vi "final_usrp_transceiver_webcam.vi"() -> ()   [LabVIEW 2014]
uses:
  <vilib>/userdefined/High Color/IMAQdx.ctl
  <vilib>/addons/Modulation/Analog/support/mod_Set Error Source.vi
  var_stop.vi
  <vilib>/addons/Modulation/Digital/Support/Common/Validators/mod_Generate Filter Coefficients Validate.vi
  <vilib>/addons/Modulation/Digital/General/subVIs/mod_Generate Filter Coefficients.vi
  <vilib>/measure/maspectr.llb/FFT Power Spectrum and PSD for 1 Chan (CDB).vi
  <vilib>/addons/Modulation/Digital/General/MT Apply Matched Filter (Generic).vi
  <vilib>/addons/Modulation/Digital/General/MT Align to Ideal Symbols (Generic).vi
  <instrlib>/niUSRP/niUSRP Fetch Rx Data (CDB Cluster).vi
  <instrlib>/niUSRP/niUSRP Write Tx Data (CDB Cluster).vi
  <vilib>/addons/Modulation/Digital/General/MT Apply Pulse Shaping Filter (Generic).vi
  <vilib>/addons/Modulation/niDMT.lvlib
  <vilib>/measure/NI_MAPro.lvlib
  <vilib>/vision/driver/NI_Vision_Acquisition_Software.lvlib
panel:
  out "error out":errorcluster
  in  "cam":T1
  in  "frame buffer size":i32=20
  in  "Stop":bool
  in  "energy threshold":dbl=-33.0 format="%#_13g"
  out "elements in frame buffer 2":i32
  out "elements in frame buffer":i32
  out "valid frames":i32
  out "elements in send buffer":i32
  in  "packet size":i32=12800
  in  "Quality (0-1000)":i32=100 caption="Quality (750)"
  out "size(s) 4":i32
  out "frame num":u32
  out "length":i32[](array[numeric])
  out "start index":i32[](array[numeric])
  out "Numeric":i32
  out "size(s) 3":i32
  out "# elements in queue 2":i32
  out "size(s) 2":i32
  out "size(s)":i32[](array[numeric])
  out "image":T2(plugin-control)
  in  "Transmit power (db)":dbl
  out "found?":bool
  out "# elements in queue":i32
  out "valid?":bool
  in  "Gray code?":bool=TRUE
  in  "Modulation":enum16{"PSK", "QAM"}(ring)
  out "packet len":u32
  in  "filter length (symbols)":i32=8
  in  "filter parameter":dbl=0.5 format="%.2f"
  in  "pulse shaping filter (none)":T3(ring)=enum."Raised Cosine"
  in  "M-PSK (4)":i32=4 caption="M-ARY"
  in  "samples per symbol (16)":i32=4
  out "packet bits length":i32
  in  "number of samples":i64=40000
  out "RX coerced gain":dbl format="%#_6f"
  out "RX coerced carrier frequency":dbl=915000000.0 format="%#_6p"
  out "RX coerced IQ rate":dbl=4000000.0 format="%#_6p"
  in  "RX active antenna":string="RX2"
  in  "RX gain":dbl format="%#_6f"
  in  "RX device names":refnum<k15>="192.168.10.2"
  out "TX coerced gain":dbl format="%#_6f"
  out "TX coerced carrier frequency":dbl=915000000.0 format="%#_6p"
  out "coerced IQ rate":dbl=4000000.0 format="%#_6p"
  in  "TX device names":refnum<k15>="192.168.10.2"
  in  "TX gain":dbl format="%#_6f"
  in  "carrier frequency":dbl=915000000.0 format="%#_6p"
  in  "IQ rate":dbl=800000.0 format="%#_6p"
  in  "stop":bool
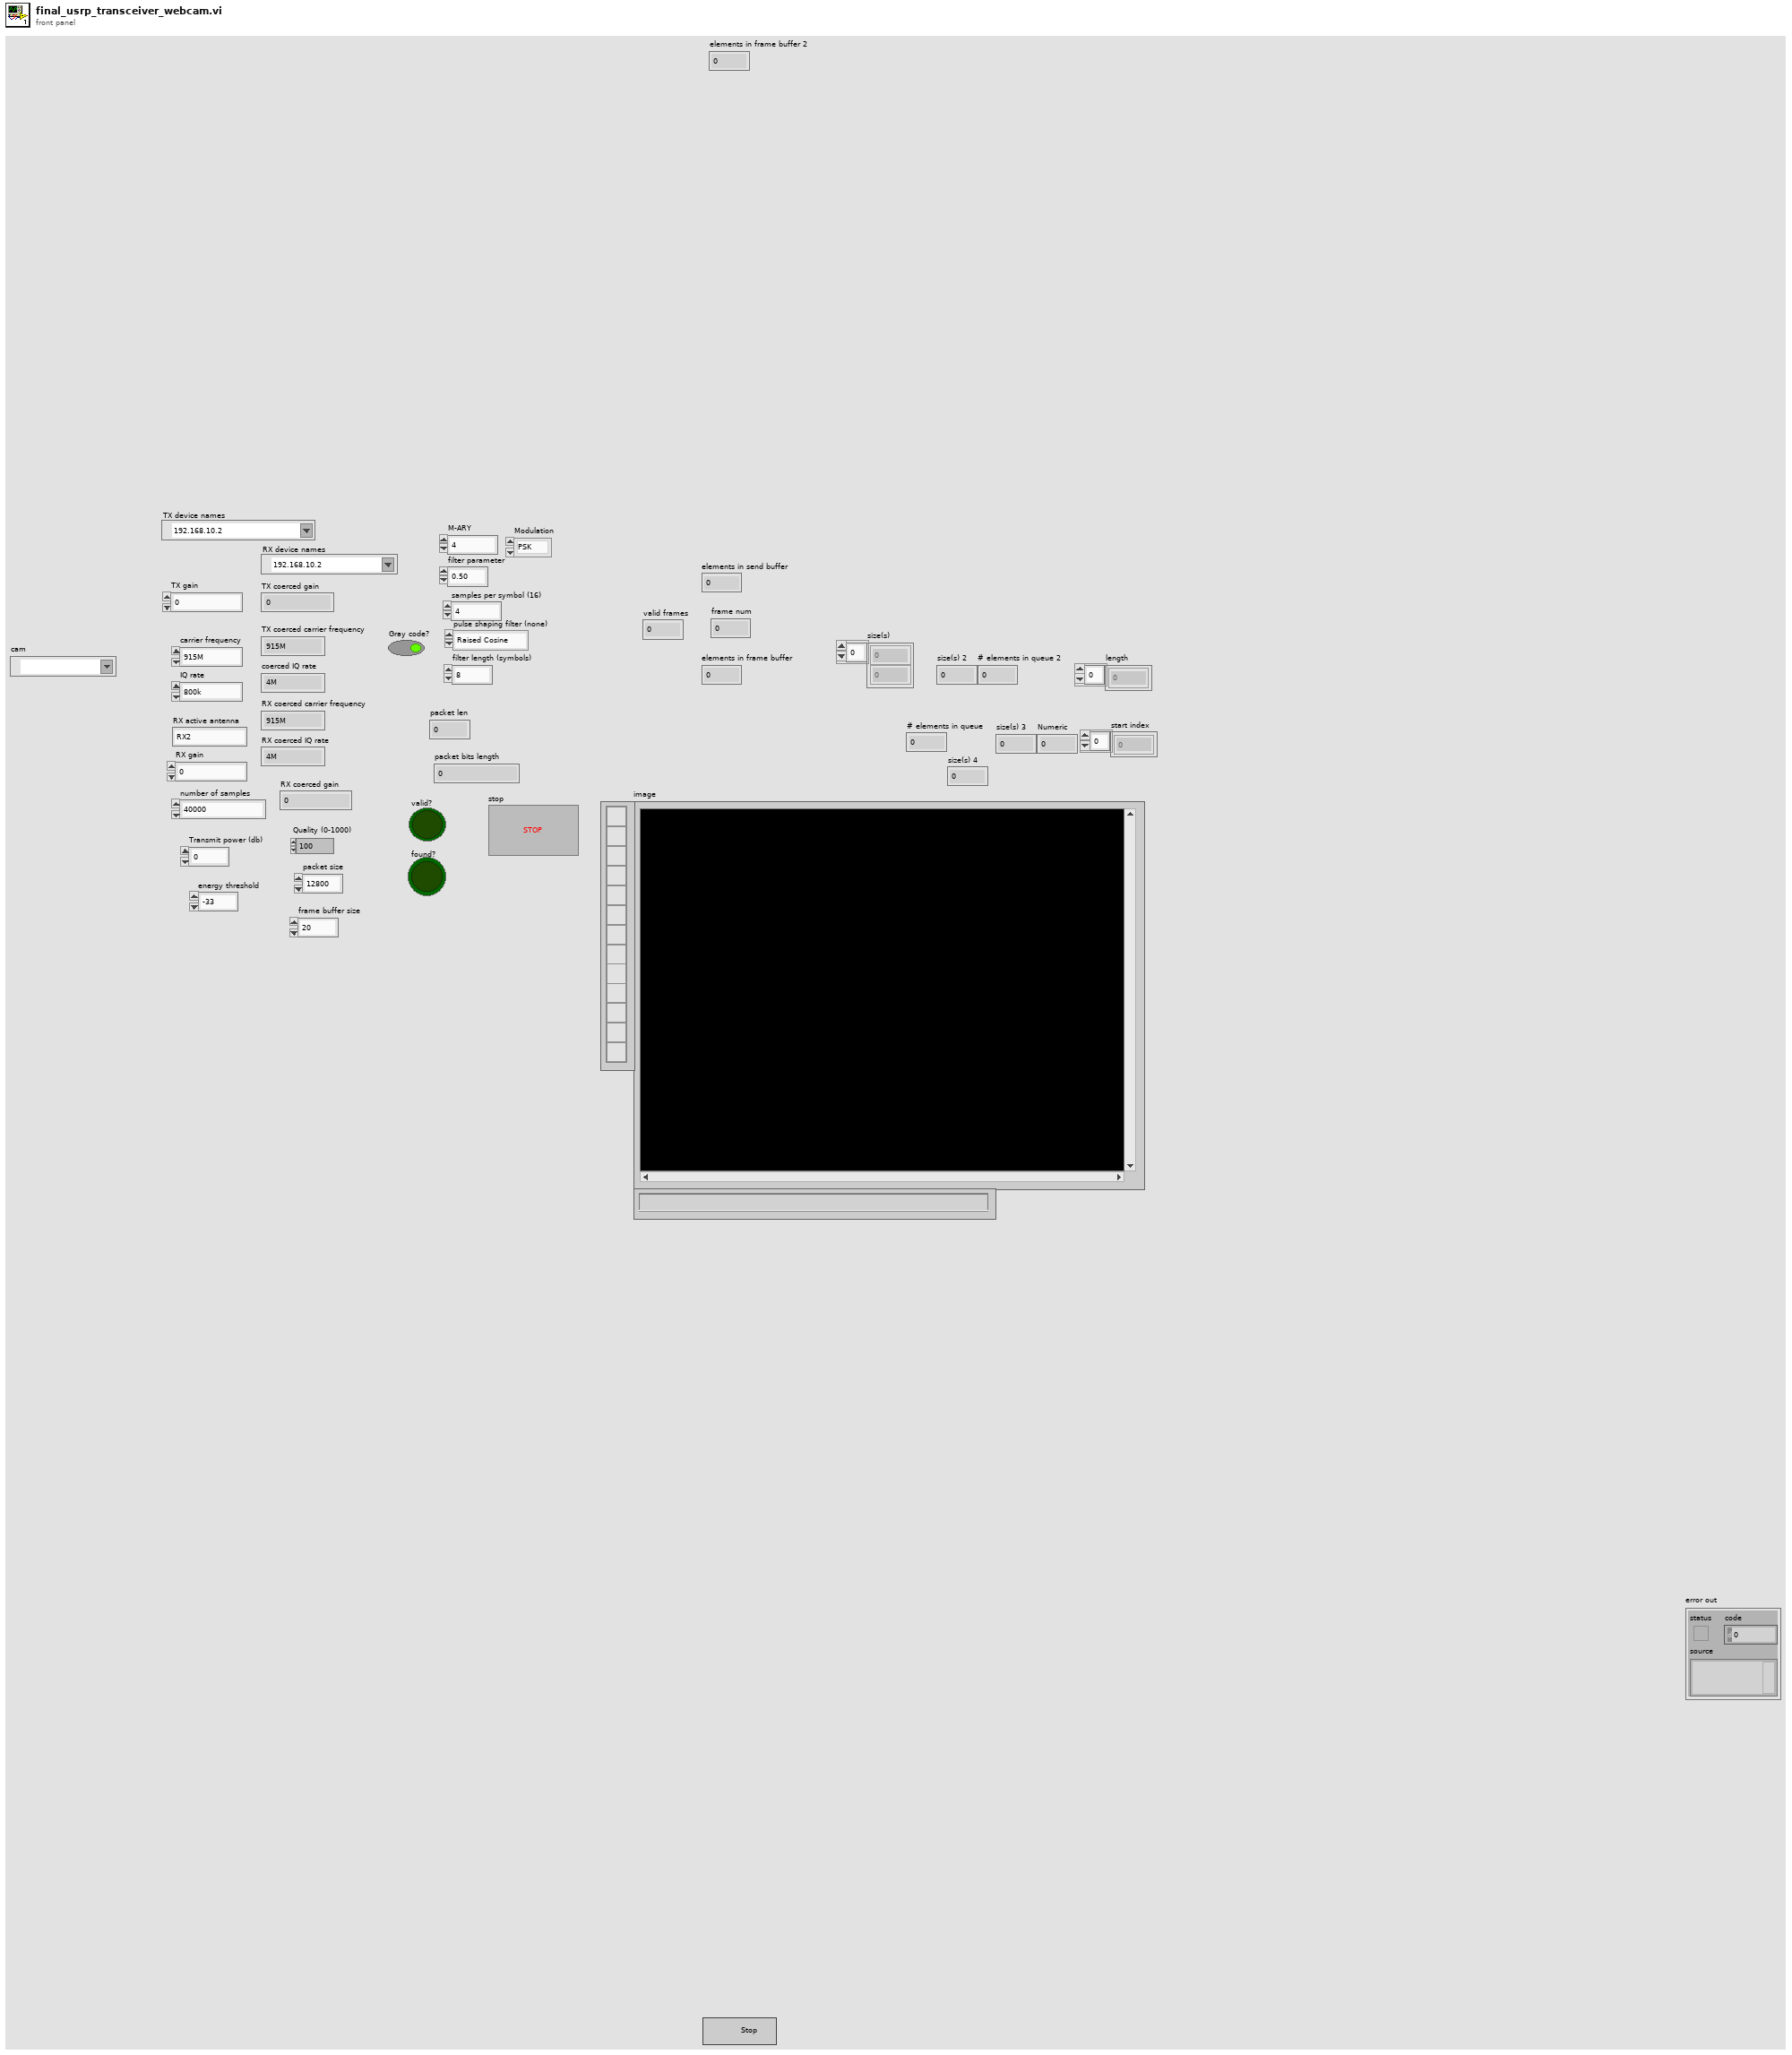
[diagram p1: front panel]
types:
  T1 = typedef "IMAQdx.ctl" = refnum<k21>
  T2 = typedef "IMAQ Image.ctl" = refnum<image>
  T3 = enum16{"none", "Raised Cosine", "Root Raised Cos", "Gaussian"}
  T4 = typedef "Image Type" = u32
  T5 = enum16{"FSK", "PSK", "QAM", "MSK", "PAM", "ASK", "CPM"}
  T6 = cluster{"samples per symbol (16)":i32, "symbol map":cdb[], "index map":u32[]}
  T7 = cluster{"samples per symbol (16)":i32, "symbol map":cdb[], i32[]}
  T8 = typedef "niAMT.lvlib/Complex Data Waveform.ctl" = cluster{"t0":dbl, "dt":dbl, "Y":cdb[]}
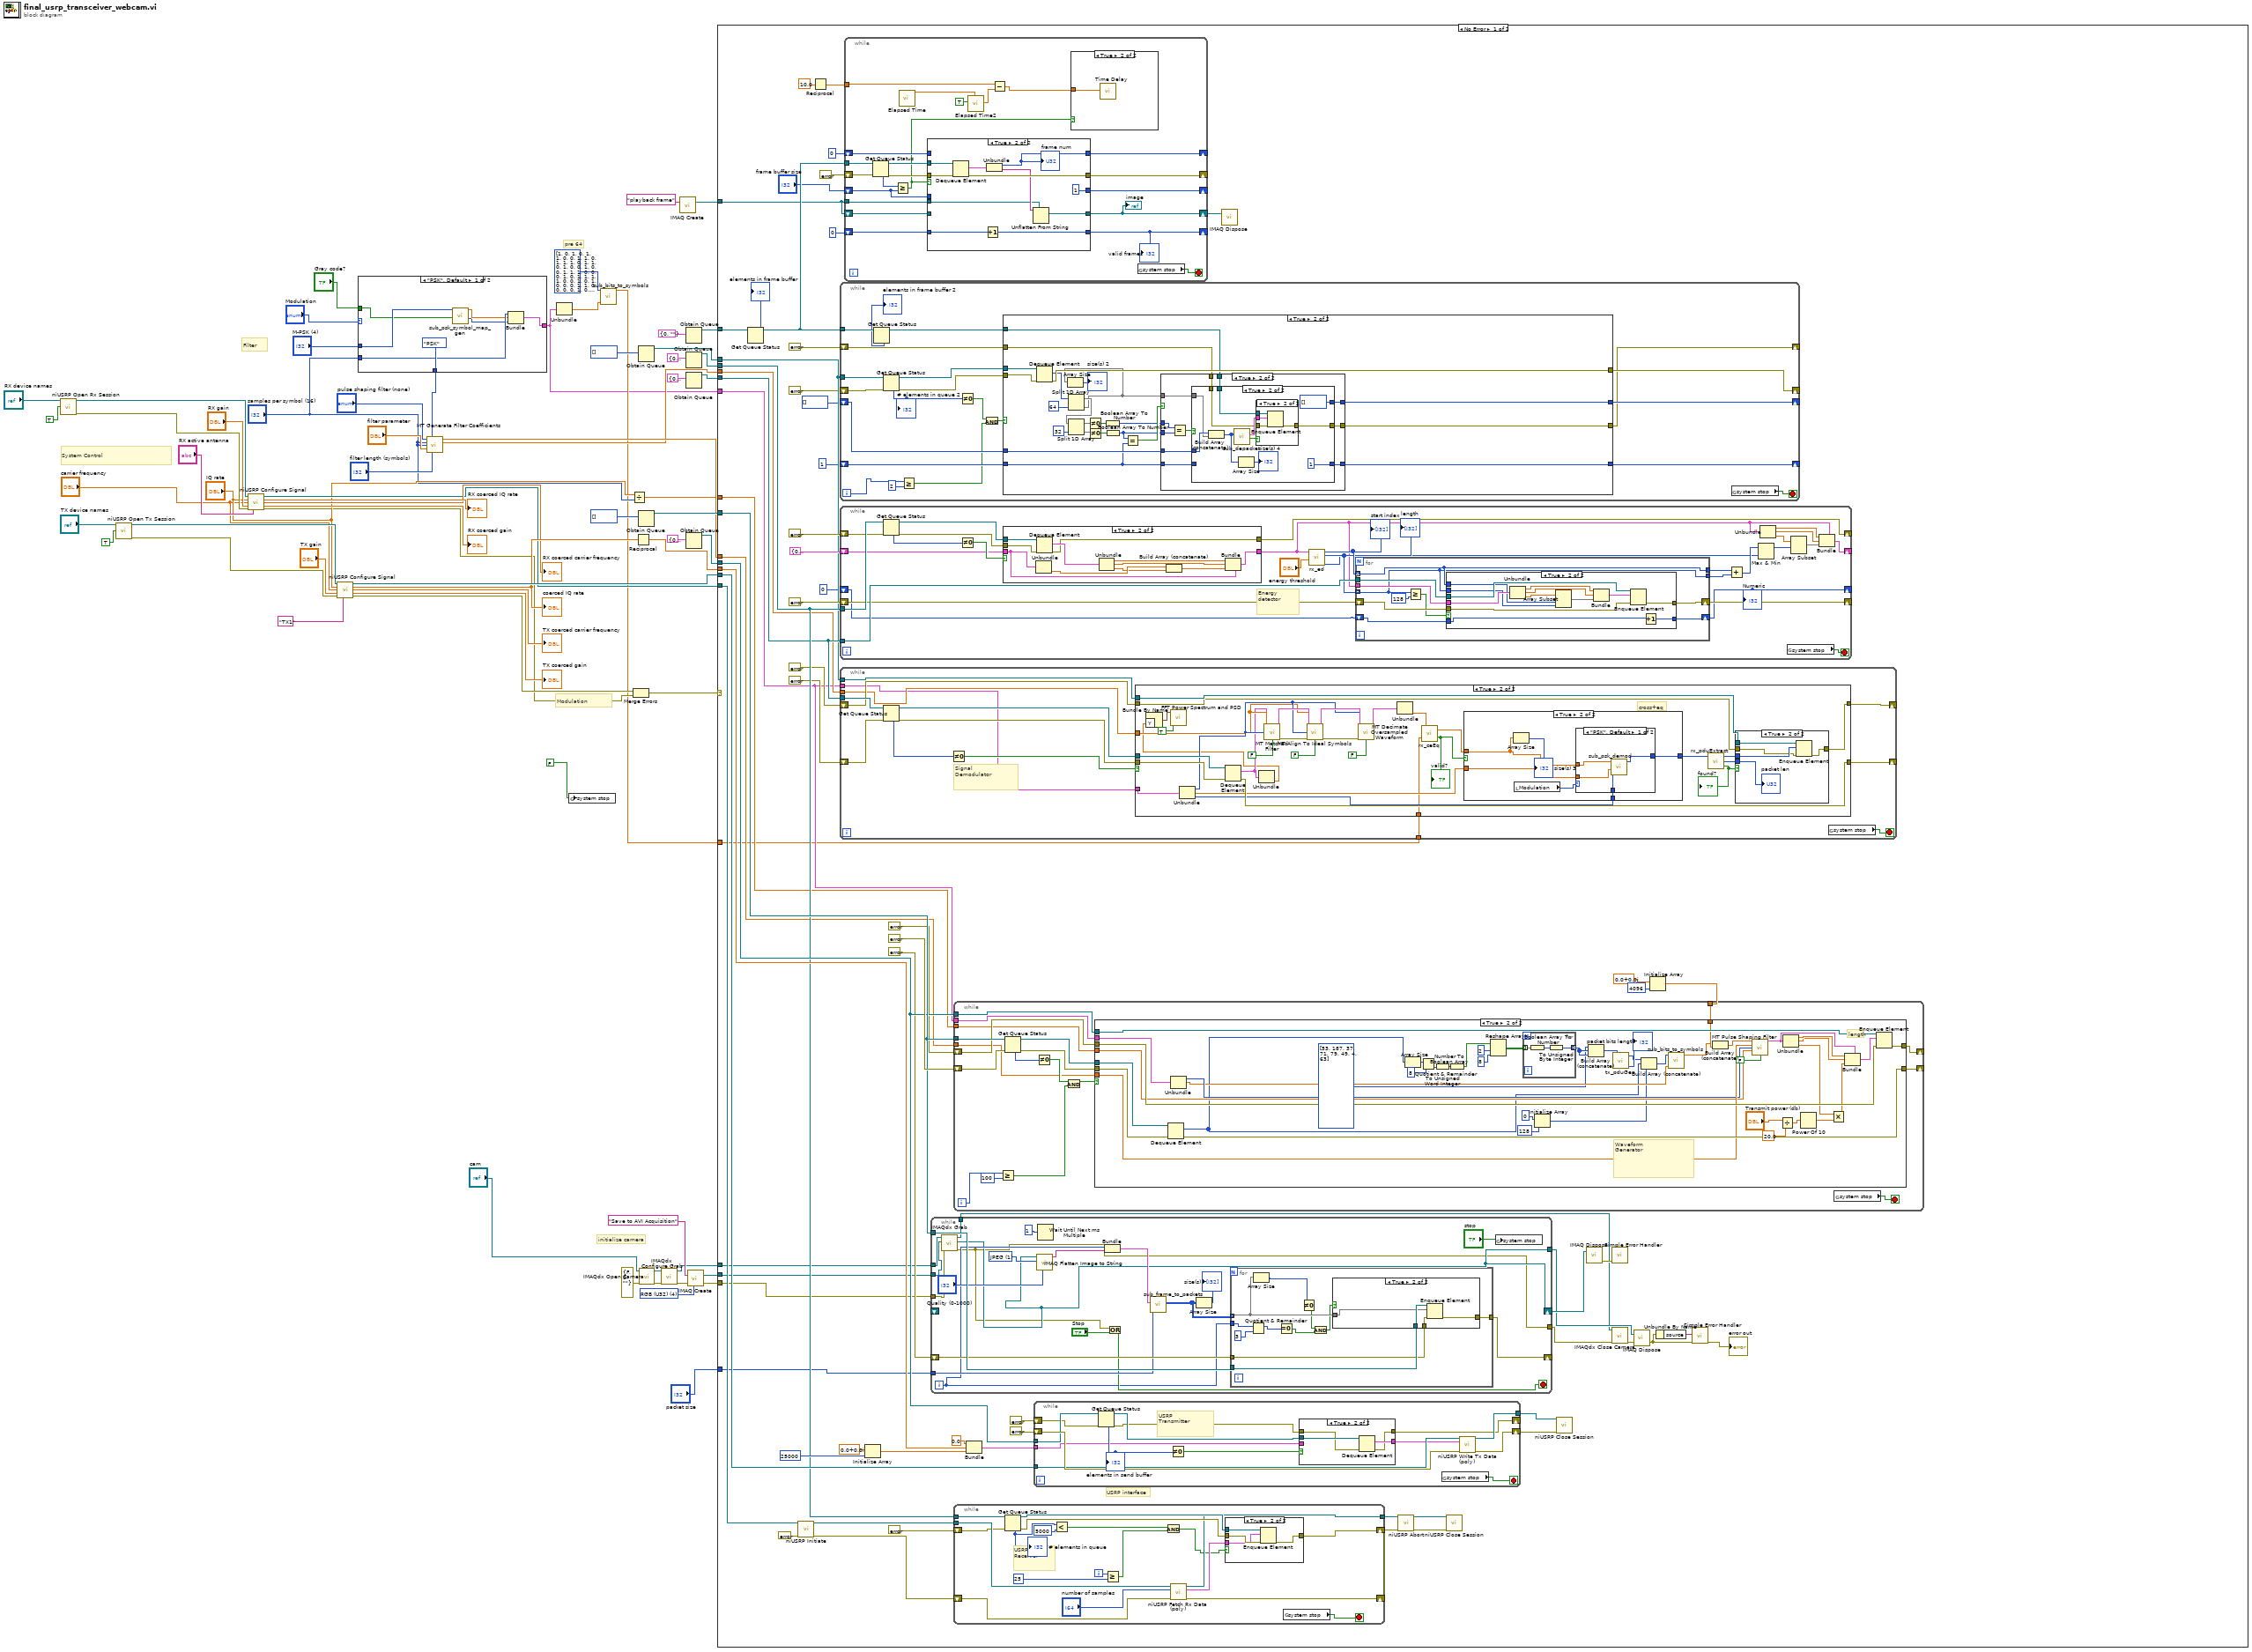
[diagram p0: block diagram]
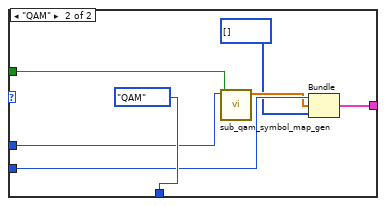
[diagram p2: hidden frame]
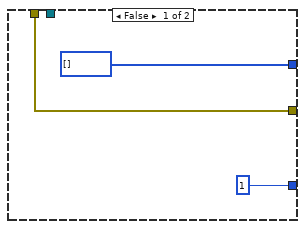
[diagram p7: hidden frame]
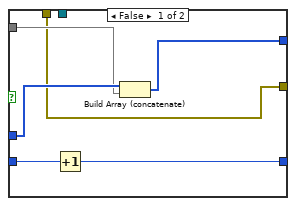
[diagram p8: hidden frame]
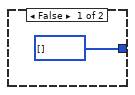
[diagram p11: hidden frame]
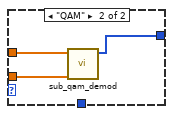
[diagram p12: hidden frame]
diagram:
  w10 = T4 4 items=["Grayscale (U8)", "Grayscale (I16)", "Grayscale (SGL)", "Complex (CSG)", "RGB (U32)", "HSL (U32)", "RGB (U64)", "Grayscale (U16)"] ("Image Type")
  # "initialize camera"
  # "pre 64"
  # "Modulation"
  # "Filter"
  # "System Control"
  n1 = call <instrlib>:"niUSRP Open Rx Session.vi"("device names"="RX device names", "reset"=TRUE) -> ("session handle out"=w53:refnum<k15>, "error out"=w52:errorcluster)  [unwired: 12 in]
  n2 = call <instrlib>:"niUSRP Open Tx Session.vi"("device names"="TX device names", "reset"=TRUE) -> ("session handle out"=w66:refnum<k15>, "error out"=w65:errorcluster)  [unwired: 12 in]
  n3 = call <instrlib>:"niUSRP Configure Signal.vi"("session handle"=w53, "IQ rate"="IQ rate", "carrier frequency"="carrier frequency", "gain"="RX gain", "error in (no error)"=w52, "active antenna"="RX active antenna") -> ("session handle out"=w44:refnum<k15>, "coerced IQ rate"=→"RX coerced IQ rate":dbl, "coerced carrier frequency"=→"RX coerced carrier frequency":dbl, "coerced gain"=→"RX coerced gain":dbl, "error out"=w28:errorcluster)  [unwired: 5 in]
  n4 = call <instrlib>:"niUSRP Configure Signal.vi"("session handle"=w66, "IQ rate"="IQ rate", "carrier frequency"="carrier frequency", "gain"="TX gain", "error in (no error)"=w65, "active antenna"="TX1") -> ("session handle out"=w57:refnum<k15>, "coerced IQ rate"=w55:dbl, "coerced carrier frequency"=→"TX coerced carrier frequency":dbl, "coerced gain"=→"TX coerced gain":dbl, "error out"=w29:errorcluster)  [unwired: 5 in]
  "coerced IQ rate" <- w55
  n5 = case shown="\"PSK\", Default" "Modulation" {
    tunnel: [T5."PSK" ("modulation type") T5."QAM" ("modulation type")] -> w23
    tunnel: "M-PSK (4)" -> [w73 w79]
    tunnel: "Gray code?" -> [w72 w80]
    tunnel: "samples per symbol (16)" -> [w71 w78]
    tunnel: [w68 w75] -> w16
    frame "PSK", Default {
      n6 = call "sub_psk_symbol_map_gen.vi"("Gray code?"=w72, "M-PSK"=w73) -> ("index map"=w69:u32[], "symbol map"=w70:cdb[])  [unwired: 8 in]
      n7 = Bundle("samples per symbol (16)"=w71, "symbol map"=w70, "index map"=w69) -> (w68:T6)  [unwired: 1 in]
    }
    frame "QAM" {
      n8 = call "sub_qam_symbol_map_gen.vi"("Gray code?"=w80, "M-QAM"=w79) -> ("symbol map"=w77:cdb[])  [unwired: 9 in]
      n9 = Bundle("samples per symbol (16)"=w78, "symbol map"=w77, i32[] []) -> (w75:T7)  [unwired: 1 in]
    }
  }
  n10 = call <vilib>:"MT Generate Filter Coefficients.vi"("pulse shaping filter (none)"="pulse shaping filter (none)", "modulation type"=w23, "pulse shaping samples per symbol (16)"="samples per symbol (16)", "matched samples per symbol (16)"="samples per symbol (16)", "filter parameter"="filter parameter", "filter length (symbols)"="filter length (symbols)") -> ("pulse shaping filter coefficients"=w34:dbl[], "matched filter coefficients"=w32:dbl[])  [unwired: 7 in, 1 out]
  n11 = Unbundle(w16) -> ("symbol map"=w18:cdb[])  [unwired: 2 out]
  n12 = global write "var_stop.vi" "system stop"(FALSE) -> ()
  n13 = call "sub_bits_to_symbols.vi"("symbol map"=w18, "bits"=i16[] [1, 0, 1, 0, 1, 1, 0, 0, 1, 1, 0, 1, 1, 1, 0, 1, 1, 0, 1, 0, 0, 1, 0, 0, 1, 1, 1, 0, 0, 0, 1, 0, 1, 1, 1, 1, 0, 0, 1, 0, 1, 0, 0, 0, 1, 1, 0, 0, 0, 0, 1, 0, 0, 0, 0, 0, 1, 1, 1, 1, 1, 1, 0, 0] ("preamble(64) 2")) -> ("symbols"=w17:cdb[])  [unwired: 9 in]
  n14 = Divide(x="IQ rate", y="samples per symbol (16)") -> (x/y=w33:dbl)
  n15 = Merge Errors(w29, w28) -> (w27:errorcluster)
  n16 = Reciprocal(x=w55) -> (1/x=w54:dbl)
  n17 = Obtain Queue(element data type=i8[] [] ("output bit stream")) -> (queue out=w39:refnum<queue>)  [unwired: 4 in, 2 out]
  n18 = Obtain Queue(element data type=i16[] []) -> (queue out=w67:refnum<queue>)  [unwired: 4 in, 2 out]
  n19 = call <vilib>:"IMAQdx Open Camera.vi"("error in"=errorcluster {"status"=FALSE, "code"=0, "source"=""}, "Session In"="cam") -> ("error out"=w6:errorcluster, "Session Out"=w8:T1)  [unwired: 8 in]
  n20 = call <vilib>:"IMAQdx Configure Grab.vi"("error in"=w6, "Session In"=w8) -> ("error out"=w5:errorcluster, "Session Out"=w3:T1)  [unwired: 8 in]
  n21 = call "IMAQ Create"("Image Name"="playback frame") -> ("New Image"=w11:T2)  [unwired: 3 in, 2 out]
  n22 = Obtain Queue(element data type=cluster{u32, "string":string} {0, "string"=""} ("frame")) -> (queue out=w14:refnum<queue>)  [unwired: 4 in, 2 out]
  n23 = Obtain Queue(element data type=cluster{"t0":dbl, "dt":dbl, "Y":cdb[]} {"t0"=0.0, "dt"=0.0, "Y"=[]} ("data")) -> (queue out=w43:refnum<queue>)  [unwired: 4 in, 2 out]
  n24 = Obtain Queue(element data type=cluster{"t0":dbl, "dt":dbl, "Y":cdb[]} {"t0"=0.0, "dt"=0.0, "Y"=[]} ("data")) -> (queue out=w40:refnum<queue>)  [unwired: 4 in, 2 out]
  n25 = Obtain Queue(element data type=cluster{"t0":dbl, "dt":dbl, "Y":cdb[]} {"t0"=0.0, "dt"=1.0, "Y"=[]} ("data")) -> (queue out=w58:refnum<queue>)  [unwired: 4 in, 2 out]
  n26 = call "IMAQ Create"("Image Name"="Save to AVI Acquisition", "Image Type"=w10, "error in (no error)"=w5) -> ("New Image"=w4:T2, "error out"=w2:errorcluster)  [unwired: 2 in]
  n27 = case shown="No Error" w27 {
    tunnel: w67 -> [w150 _]
    tunnel: w58 -> [w145 _]
    tunnel: w57 -> [w146 _]
    tunnel: w54 -> [w139 _]
    tunnel: w44 -> [w134 _]
    tunnel: w43 -> [w128 _]
    tunnel: w40 -> [w124 _]
    tunnel: w39 -> [w122 _]
    tunnel: w16 -> [w116 _]
    tunnel: w34 -> [w119 _]
    tunnel: w33 -> [w118 _]
    tunnel: w32 -> [w117 _]
    tunnel: w17 -> [w110 _]
    tunnel: w14 -> [w106 _]
    tunnel: "packet size" -> [w100 _]
    tunnel: w11 -> [w92 _]
    tunnel: w4 -> [w91 _]
    tunnel: w3 -> [w90 _]
    tunnel: w2 -> [w89 _]
    frame No Error {
      # "USRP interface"
      n28 = Get Queue Status(queue=w106) -> (queue out=w98:refnum<queue>, # elements in queue=→"elements in frame buffer":i32)  [unwired: 2 in, 6 out]
      n29 = call <instrlib>:"niUSRP Initiate.vi"("session handle"=w134, "error in (no error)"=errorcluster {"status"=FALSE, "code"=0, "source"=""}) -> ("session handle out"=w133:refnum<k15>, "error out"=w132:errorcluster)  [unwired: 12 in]
      n30 = Reciprocal(x=10.0) -> (1/x=w101:dbl)
      n31 = while {
        tunnel: w122 -> [w248]
        shift-right: [w241] -> _
        shift-left: errorcluster {"status"=FALSE, "code"=0, "source"=""} ("error out") -> [w247]
        shift-right: [w239] -> _
        shift-left: u32 1 -> [w240]
        shift-right: [w238] -> _
        shift-left: i8[] [] ("second subarray") -> [w237]
        tunnel: w98 -> [w236]
        shift-right: [w234] -> _
        shift-left: errorcluster {"status"=FALSE, "code"=0, "source"=""} ("error out") -> [w235]
        i -> [w232]
        stop <- w246 stop-if-true
        n32 = Get Queue Status(queue=w236) -> (queue out=w229:refnum<queue>, # elements in queue=→"elements in frame buffer 2":i32)  [unwired: 2 in, 6 out]
        n33 = Get Queue Status(queue=w248, error in (no error)=w247) -> (queue out=w243:refnum<queue>, error out=w242:errorcluster, # elements in queue=w245:i32)  [unwired: 1 in, 5 out]
        "# elements in queue 2" <- w245
        n34 = Greater Or Equal?(x=w232, y=2) -> (x >= y?=w231:bool)
        n35 = Not Equal To 0?(x=w245) -> (x != 0?=w244:bool)
        n36 = And(x=w244, y=w231) -> (x .and. y?=w230:bool)
        n37 = case shown="True" w230 {
          tunnel: w243 -> [_ w275]
          tunnel: w242 -> [w252 w274]
          tunnel: [w252 w273] -> w241
          tunnel: w240 -> [w251 w259]
          tunnel: [w251 w260] -> w239
          tunnel: [w249 w264] -> w238
          tunnel: w237 -> [w249 w261]
          tunnel: w229 -> [_ w258]
          tunnel: w235 -> [w250 w257]
          tunnel: [w250 w256] -> w234
          frame False {
          }
          frame True {
            n38 = Dequeue Element(queue=w275, error in (no error)=w274) -> (element=w255:i8[], error out=w273:errorcluster)  [unwired: 1 in, 2 out]
            n39 = Split 1D Array(array=w255, index=64) -> (first subarray=w266:i8[], second subarray=w253:i8[])
            n40 = Array Size(array=w253) -> (size(s)=→"size(s) 2":i32)
            n41 = Split 1D Array(array=w266, index=32) -> (first subarray=w269:i8[], second subarray=w270:i8[])
            n42 = Not Equal To 0?(x=w269) -> (x != 0?=w268:bool[])
            n43 = Not Equal To 0?(x=w270) -> (x != 0?=w267:bool[])
            n44 = Boolean Array To Number(Boolean array=w268) -> (number=w263:u32)
            n45 = Boolean Array To Number(Boolean array=w267) -> (number=w262:u32)
            n46 = Equal?(x=w262, y=w259) -> (x = y?=w265:bool)
            n47 = case shown="True" w265 {
              tunnel: [i8[] [] ("second subarray") w286] -> w264
              tunnel: w263 -> [_ w289]
              tunnel: w262 -> [_ w288]
              tunnel: w261 -> [_ w285]
              tunnel: w253 -> [_ w284]
              tunnel: [u32 1 w283] -> w260
              tunnel: w259 -> [_ w282]
              tunnel: w258 -> [_ w281]
              tunnel: w257 -> [w276 w280]
              tunnel: [w276 w279] -> w256
              frame False {
              }
              frame True {
                n48 = Equal?(x=w289, y=w288) -> (x = y?=w287:bool)
                n49 = case shown="True" w287 {
                  tunnel: [w293 i8[] [] ("second subarray")] -> w286
                  tunnel: w285 -> [w295 w304]
                  tunnel: w284 -> [w294 w303]
                  tunnel: [w291 u32 1] -> w283
                  tunnel: w282 -> [w292 _]
                  tunnel: w281 -> [_ w302]
                  tunnel: w280 -> [w290 w300]
                  tunnel: [w290 w299] -> w279
                  frame False {
                    n50 = Increment(x=w292) -> (x+1=w291:u32)
                    n51 = Build Array (concatenate)(w295, w294) -> (w293:i8[])
                  }
                  frame True {
                    n52 = Build Array (concatenate)(w304, w303) -> (w298:i8[])
                    n53 = call "sub_depacket.vi"("bitstream"=w298) -> ("CRC valid"=w296:bool, "frame"=w301:cluster{u32, "string":string})  [unwired: 9 in]
                    n54 = Array Size(array=w298) -> (size(s)=→"size(s) 4":i32)
                    n55 = case shown="True" w296 {
                      tunnel: w302 -> [_ w311]
                      tunnel: w301 -> [_ w310]
                      tunnel: w300 -> [w307 w309]
                      tunnel: [w307 w308] -> w299
                      frame False {
                      }
                      frame True {
                        n56 = Enqueue Element(queue=w311, element=w310, error in (no error)=w309) -> (error out=w308:errorcluster)  [unwired: 1 in, 2 out]
                      }
                    }
                  }
                }
              }
            }
          }
        }
        n57 = global read "var_stop.vi" "system stop"() -> (w246:bool)
      }
      n58 = while {
        tunnel: w128 -> [w406]
        shift-right: [w399] -> _
        shift-left: errorcluster {"status"=FALSE, "code"=0, "source"=""} ("error out") -> [w405]
        shift-right: [w385] -> _
        shift-left: cluster{"t0":dbl, "dt":dbl, "Y":cdb[]} {"t0"=0.0, "dt"=0.0, "Y"=[]} ("data") -> [w400]
        tunnel: w124 -> [w398]
        shift-right: [w397] -> _
        shift-left: errorcluster {"status"=FALSE, "code"=0, "source"=""} ("error out") -> [w396]
        shift-right: [w380] -> _
        shift-left: 0 -> [w381]
        stop <- w395 stop-if-true
        # "Energy\ndetector"
        n59 = Get Queue Status(queue=w406, error in (no error)=w405) -> (queue out=w401:refnum<queue>, error out=w402:errorcluster, # elements in queue=w404:i32)  [unwired: 1 in, 5 out]
        n60 = Not Equal To 0?(x=w404) -> (x != 0?=w403:bool)
        n61 = case shown="True" w403 {
          tunnel: w402 -> [w433 w444]
          tunnel: w401 -> [_ w443]
          tunnel: w400 -> [w432 w438]
          tunnel: [w433 w435] -> w399
          tunnel: [w432 w434] -> w392
          frame False {
          }
          frame True {
            n62 = Unbundle(w438) -> ("Y"=w441:cdb[])  [unwired: 2 out]
            n63 = Dequeue Element(queue=w443, error in (no error)=w444) -> (element=w442:cluster{"t0":dbl, "dt":dbl, "Y":cdb[]}, error out=w435:errorcluster)  [unwired: 1 in, 2 out]
            n64 = Unbundle(w442) -> ("t0"=w437:dbl, "dt"=w436:dbl, "Y"=w440:cdb[])
            n65 = Build Array (concatenate)(w441, w440) -> (w439:cdb[])
            n66 = Bundle(cluster=w438, "t0"=w437, "dt"=w436, "Y"=w439) -> (w434:cluster{"t0":dbl, "dt":dbl, "Y":cdb[]})
          }
        }
        n67 = call "rx_ed.vi"("energy threshold"="energy threshold", "Wavefrom"=w392) -> ("first pulse"=w382:i32, "length"=w393:i32[], "start index"=w394:i32[])  [unwired: 7 in]
        "start index" <- w394
        "length" <- w393
        n68 = for {
          tunnel: w398 -> [w416]
          tunnel: w392 -> [w413]
          shift-right: [w415] -> w397
          shift-left: w396 -> [w414]
          tunnel: w394 -> [w412] mode=indexing
          tunnel: w393 -> [w411] mode=indexing
          tunnel: [w412] -> w388
          tunnel: [w411] -> w387
          shift-right: [w407] -> w380
          shift-left: w381 -> [w408]
          n69 = Greater Or Equal?(x=w411, y=128) -> (x >= y?=w409:bool)
          n70 = case shown="True" w409 {
            tunnel: w416 -> [_ w431]
            tunnel: [w418 w430] -> w415
            tunnel: w414 -> [w418 w429]
            tunnel: w413 -> [_ w428]
            tunnel: w412 -> [_ w422]
            tunnel: w411 -> [_ w421]
            tunnel: w408 -> [w417 w420]
            tunnel: [w417 w419] -> w407
            frame False {
            }
            frame True {
              n71 = Unbundle(w428) -> ("t0"=w426:dbl, "dt"=w427:dbl, "Y"=w424:cdb[])
              n72 = Array Subset(array=w424, index=w422, length=w421) -> (w423:cdb[])
              n73 = Bundle("t0"=w426, "dt"=w427, w423) -> (w425:cluster{"t0":dbl, "dt":dbl, cdb[]})  [unwired: 1 in]
              n74 = Enqueue Element(queue=w431, element=w425, error in (no error)=w429) -> (error out=w430:errorcluster)  [unwired: 1 in, 2 out]
              n75 = Increment(x=w420) -> (x+1=w419:i32)
            }
          }
        }
        "Numeric" <- w380
        n76 = Add(x=w388, y=w387) -> (x+y=w384:i32)
        n77 = Max & Min(x=w384, y=w382) -> (max(x,y)=w383:i32)  [unwired: 1 out]
        n78 = Unbundle(w392) -> ("t0"=w391:dbl, "dt"=w390:dbl, "Y"=w389:cdb[])
        n79 = global read "var_stop.vi" "system stop"() -> (w395:bool)
        n80 = Array Subset(array=w389, index=w383) -> (w386:cdb[])  [unwired: 1 in]
        n81 = Bundle(cluster=w392, "t0"=w391, "dt"=w390, "Y"=w386) -> (w385:cluster{"t0":dbl, "dt":dbl, "Y":cdb[]})
      }
      n82 = while {
        tunnel: w124 -> [w325]
        shift-right: [w319] -> _
        shift-left: errorcluster {"status"=FALSE, "code"=0, "source"=""} ("error out") -> [w324]
        tunnel: w122 -> [w318]
        shift-right: [w317] -> _
        shift-left: errorcluster {"status"=FALSE, "code"=0, "source"=""} ("error out") -> [w316]
        tunnel: w117 -> [w314]
        tunnel: w116 -> [w313]
        tunnel: w110 -> [w312]
        stop <- w315 stop-if-true
        # "Signal \nDemodulator"
        n83 = Get Queue Status(queue=w325, error in (no error)=w324) -> (queue out=w321:refnum<queue>, error out=w320:errorcluster, # elements in queue=w323:i32)  [unwired: 1 in, 5 out]
        n84 = Not Equal To 0?(x=w323) -> (x != 0?=w322:bool)
        n85 = case shown="True" w322 {
          tunnel: w321 -> [_ w357]
          tunnel: w320 -> [w327 w358]
          tunnel: [w327 w356] -> w319
          tunnel: w318 -> [_ w346]
          tunnel: [w326 w345] -> w317
          tunnel: w316 -> [w326 w344]
          tunnel: w314 -> [_ w333]
          tunnel: w313 -> [_ w337]
          tunnel: w312 -> [_ w330]
          frame False {
          }
          frame True {
            # "cross+eq"
            n86 = Unbundle(w337) -> ("samples per symbol (16)"=w336:i32, "symbol map"=w335:cdb[], "index map"=w334:u32[])
            n87 = Dequeue Element(queue=w357, error in (no error)=w358) -> (element=w329:cluster{"t0":dbl, "dt":dbl, "Y":cdb[]}, error out=w356:errorcluster)  [unwired: 1 in, 2 out]
            n88 = Unbundle(w329) -> ("Y"=w328:cdb[])  [unwired: 2 out]
            n89 = Bundle By Name("Y"=w328) -> (w332:waveform(cdb))  [unwired: 1 in]
            n90 = call-poly <vilib>:"FFT Power Spectrum and PSD.vi"("dB On (F)"=TRUE, "time signal"=w332) -> ()  [unwired: 6 in, 4 out]
            n91 = call-poly <vilib>:"MT Matched Filter.vi"("input complex waveform"=w329, "matched filter coefficients"=w333, "samples per symbol (16)"=w336, "reset? (T)"=FALSE) -> ("output complex waveform"=w355:T8, "error out"=w354:errorcluster)  [unwired: 10 in]
            n92 = call-poly <vilib>:"MT Align To Ideal Symbols.vi"("input complex waveform"=w355, "matched filter coefficients"=w333, "samples per symbol (16)"=w336, "error in (no error)"=w354, "reset? (T)"=FALSE) -> ("output complex waveform"=w352:T8, "error out"=w353:errorcluster)  [unwired: 8 in, 1 out]
            n93 = call <vilib>:"MT Decimate Oversampled Waveform.vi"("input complex waveform"=w352, "decimation factor"=w336, "error in (no error)"=w353, "reset? (T)"=FALSE) -> ("output complex waveform"=w351:T8)  [unwired: 10 in, 1 out]
            n94 = Unbundle(w351) -> ("Y"=w347:cdb[])  [unwired: 2 out]
            n95 = call "rx_ceEq.vi"("preamble"=w330, "symbols"=w347) -> ("valid?"=w342:bool, "eq symbols"=w343:cdb[])
            "valid?" <- w342
            n96 = case shown="True" w342 {
              tunnel: [i8[] [] ("output bit stream") w363] -> w350
              tunnel: w335 -> [_ w364]
              tunnel: w343 -> [_ w361]
              tunnel: w334 -> [_ w362]
              frame False {
              }
              frame True {
                n97 = Array Size(array=w361) -> (size(s)=→"size(s) 3":i32)
                n98 = local read "Modulation"() -> (w365:enum16{"PSK", "QAM"})
                n99 = case shown="\"PSK\", Default" w365 {
                  tunnel: w361 -> [w369 w372]
                  tunnel: w364 -> [w368 w371]
                  tunnel: [w366 w370] -> w363
                  tunnel: w362 -> [w367 _]
                  frame "PSK", Default {
                    n100 = call "sub_psk_demod.vi"("index map"=w367, "symbol map"=w368, "symbol"=w369) -> ("bitstream"=w366:i16[])  [unwired: 8 in]
                  }
                  frame "QAM" {
                    n101 = call "sub_qam_demod.vi"("symbol map"=w371, "symbol"=w372) -> ("bitstream"=w370:i16[])  [unwired: 9 in]
                  }
                }
              }
            }
            n102 = call "rx_pduExtract.vi"("output bit stream"=w350) -> ("found?"=w349:bool, "packet len"=w341:u32, "ppdu"=w348:i8[])  [unwired: 2 in]
            "found?" <- w349
            n103 = case shown="True" w349 {
              tunnel: w348 -> [_ w376]
              tunnel: w346 -> [_ w378]
              tunnel: [w373 w377] -> w345
              tunnel: w344 -> [w373 w374]
              tunnel: w341 -> [_ w375]
              frame False {
              }
              frame True {
                n104 = Enqueue Element(queue=w378, element=w376, error in (no error)=w374) -> (error out=w377:errorcluster)  [unwired: 1 in, 2 out]
                "packet len" <- w375
              }
            }
          }
        }
        n105 = global read "var_stop.vi" "system stop"() -> (w315:bool)
      }
      n106 = while {
        tunnel: w98 -> [w210]
        shift-right: [w206] -> _
        shift-left: errorcluster {"status"=FALSE, "code"=0, "source"=""} ("error out") -> [w209]
        shift-right: [w203] -> _
        shift-left: 0 -> [w202]
        tunnel: w101 -> [w198]
        shift-right: [w199] -> _
        shift-left: 0 -> [w200]
        shift-right: [w194] -> _
        shift-left: "frame buffer size" -> [w193]
        shift-right: [w190] -> w93
        shift-left: w92 -> [w191]
        tunnel: w92 -> [w189]
        stop <- w205 stop-if-true
        n107 = Get Queue Status(queue=w210, error in (no error)=w209) -> (queue out=w208:refnum<queue>, error out=w207:errorcluster, # elements in queue=w195:i32)  [unwired: 1 in, 5 out]
        n108 = Greater Or Equal?(x=w195, y=w193) -> (x >= y?=w192:bool)
        n109 = call "Elapsed Time"() -> ("Present (s)"=w197:dbl)  [unwired: 12 in, 7 out]
        n110 = case shown="True" w192 {
          tunnel: w208 -> [_ w227]
          tunnel: w207 -> [w216 w226]
          tunnel: [w216 w224] -> w206
          tunnel: [w215 w222] -> w203
          tunnel: w202 -> [w215 _]
          tunnel: w200 -> [w214 w221]
          tunnel: [w214 w220] -> w199
          tunnel: [w213 1] -> w194
          tunnel: w193 -> [w213 _]
          tunnel: [w212 w218] -> w190
          tunnel: w191 -> [w212 _]
          tunnel: w189 -> [_ w217]
          frame False {
          }
          frame True {
            n111 = Dequeue Element(queue=w227, error in (no error)=w226) -> (element=w225:cluster{u32, "string":string}, error out=w224:errorcluster)  [unwired: 1 in, 2 out]
            n112 = Increment(x=w221) -> (x+1=w220:i32)
            n113 = Unbundle(w225) -> (w222:u32, "string"=w223:string)
            "frame num" <- w222
            n114 = Unflatten From String(type=w217, binary string=w223) -> (value=w218:T2)  [unwired: 3 in, 2 out]
          }
        }
        "valid frames" <- w199
        "image" <- w190
        n115 = call "Elapsed Time2"("Reset"=TRUE, "Set Start Time (s)"=w197) -> ("Elapsed Time (s)"=w201:dbl)  [unwired: 10 in, 7 out]
        n116 = Subtract(x=w198, y=w201) -> (x-y=w196:dbl)
        n117 = case shown="True" w192 {
          tunnel: w196 -> [_ w211]
          frame False {
          }
          frame True {
            n118 = call "Time Delay"("Delay Time (s)"=w211) -> ()  [unwired: 10 in, 1 out]
          }
        }
        n119 = global read "var_stop.vi" "system stop"() -> (w205:bool)
      }
      n120 = Initialize Array(cdb 0.0+0.0i, 25000 ("dimension size")) -> (w140:cdb[])
      n121 = while {
        tunnel: w150 -> [w171]
        shift-right: [w169] -> _
        shift-left: errorcluster {"status"=FALSE, "code"=0, "source"=""} ("error out") -> [w170]
        tunnel: w100 -> [w165]
        tunnel: [w157] -> w84
        shift-right: [w157] -> w94
        shift-left: _ -> [_]
        tunnel: w89 -> [w154]
        tunnel: w91 -> [w155]
        tunnel: w90 -> [w156]
        tunnel: [w153] -> w83
        tunnel: [w152] -> w82
        i -> [w158]
        stop <- w159 stop-if-true
        w163 = 1 items=["None", "JPEG", "PACKED BINARY"] ("Compression (None)")
        n122 = call <vilib>:"IMAQdx Grab.vi"("error in"=w154, "Image In"=w155, "Session In"=w156) -> ("error out"=w152:errorcluster, "Image Out"=w157:T2, "Session Out"=w153:T1)  [unwired: 5 in, 1 out]
        n123 = call "IMAQ Flatten Image to String"("Quality (750)"="Quality (0-1000)", "Compression (None)"=w163, "Image"=w157) -> ("Data String"=w162:string)  [unwired: 7 in, 1 out]
        n124 = Wait Until Next ms Multiple(millisecond multiple=u32 1) -> ()  [unwired: 1 out]
        n125 = Bundle(w158, "Data String"=w162) -> (w161:cluster{i32, "Data String":string})  [unwired: 1 in]
        n126 = Or(x=w152, y="Stop") -> (x .or. y?=w159:bool)
        n127 = call "sub_frame_to_packets.vi"("packet size"=w165, "Cluster"=w161) -> ("packets"=w168:i16[][])  [unwired: 9 in]
        n128 = Array Size(array=w168) -> (size(s)=→"size(s)":i32[])
        n129 = for {
          tunnel: w171 -> [w183]
          tunnel: w170 -> [w182]
          tunnel: [w181] -> w169
          tunnel: w168 -> [w179] mode=indexing
          tunnel: w158 -> [w178]
          n130 = Quotient & Remainder(x=w178, y=3) -> (x-y*floor(x/y)=w176:i32)  [unwired: 1 out]
          n131 = Array Size(array=w179) -> (size(s)=w180:i32)
          n132 = Equal To 0?(x=w176) -> (x = 0?=w175:bool)
          n133 = Not Equal To 0?(x=w180) -> (x != 0?=w174:bool)
          n134 = And(x=w174, y=w175) -> (x .and. y?=w173:bool)
          n135 = case shown="True" w173 {
            tunnel: w179 -> [_ w185]
            tunnel: w183 -> [_ w188]
            tunnel: w182 -> [w184 w187]
            tunnel: [w184 w186] -> w181
            frame False {
            }
            frame True {
              n136 = Enqueue Element(queue=w188, element=w185, error in (no error)=w187) -> (error out=w186:errorcluster)  [unwired: 1 in, 2 out]
            }
          }
        }
        n137 = global write "var_stop.vi" "system stop"("stop") -> ()
      }
      n138 = while {
        tunnel: w133 -> [w463]
        shift-right: [w452] -> w129
        shift-left: w132 -> [w462]
        tunnel: w128 -> [w460]
        shift-right: [w454] -> _
        shift-left: errorcluster {"status"=FALSE, "code"=0, "source"=""} ("error out") -> [w459]
        tunnel: [w453] -> w130
        i -> [w450]
        stop <- w451 stop-if-true
        # "USRP\nReceiver"
        n139 = Get Queue Status(queue=w460, error in (no error)=w459) -> (queue out=w456:refnum<queue>, error out=w455:errorcluster, # elements in queue=w458:i32)  [unwired: 1 in, 5 out]
        "# elements in queue" <- w458
        n140 = Less?(x=w458, y=5000) -> (x < y?=w448:bool)
        n141 = Greater Or Equal?(x=w450, y=25) -> (x >= y?=w447:bool)
        n142 = And(x=w448, y=w447) -> (x .and. y?=w445:bool)
        n143 = call-poly <instrlib>:"niUSRP Fetch Rx Data (poly).vi"("session handle"=w463, "number of samples"="number of samples", "error in (no error)"=w462) -> ("session handle out"=w453:refnum<k15>, "data"=w446:cluster{"t0":dbl, "dt":dbl, "Y":cdb[]}, "error out"=w452:errorcluster)  [unwired: 9 in, 1 out]
        n144 = case shown="True" w445 {
          tunnel: w456 -> [_ w468]
          tunnel: w455 -> [w464 w467]
          tunnel: [w464 w466] -> w454
          tunnel: w446 -> [_ w465]
          frame False {
          }
          frame True {
            n145 = Enqueue Element(queue=w468, element=w465, error in (no error)=w467) -> (error out=w466:errorcluster)  [unwired: 1 in, 2 out]
          }
        }
        n146 = global read "var_stop.vi" "system stop"() -> (w451:bool)
      }
      n147 = Bundle(0.0, w139, w140) -> (w137:cluster{dbl, dbl, cdb[]})  [unwired: 1 in]
      n148 = while {
        shift-right: [w478] -> w149
        shift-left: errorcluster {"status"=FALSE, "code"=0, "source"=""} ("error out") -> [w476]
        tunnel: [w477] -> w148
        tunnel: w146 -> [w475]
        tunnel: w145 -> [w473]
        shift-right: [w471] -> _
        shift-left: errorcluster {"status"=FALSE, "code"=0, "source"=""} ("error out") -> [w472]
        tunnel: w137 -> [w470]
        stop <- w469 stop-if-true
        # "USRP\nTransmitter"
        n149 = Get Queue Status(queue=w473, error in (no error)=w472) -> (queue out=w480:refnum<queue>, error out=w479:errorcluster, # elements in queue=w482:i32)  [unwired: 1 in, 5 out]
        "elements in send buffer" <- w482
        n150 = Not Equal To 0?(x=w482) -> (x != 0?=w481:bool)
        n151 = case shown="True" w481 {
          tunnel: w480 -> [_ w488]
          tunnel: w479 -> [w483 w487]
          tunnel: [w484 w486] -> w474
          tunnel: [w483 w485] -> w471
          tunnel: w470 -> [w484 _]
          frame False {
          }
          frame True {
            n152 = Dequeue Element(queue=w488, error in (no error)=w487) -> (element=w486:cluster{"t0":dbl, "dt":dbl, "Y":cdb[]}, error out=w485:errorcluster)  [unwired: 1 in, 2 out]
          }
        }
        n153 = global read "var_stop.vi" "system stop"() -> (w469:bool)
        n154 = call-poly <instrlib>:"niUSRP Write Tx Data (poly).vi"("session handle"=w475, "data"=w474, "error in (no error)"=w476) -> ("session handle out"=w477:refnum<k15>, "error out"=w478:errorcluster)  [unwired: 11 in]
      }
      n155 = call "IMAQ Dispose"("Image"=w93) -> ()  [unwired: 2 in, 4 out]
      n156 = call <instrlib>:"niUSRP Abort.vi"("session handle"=w130, "error in (no error)"=w129) -> ("session handle out"=w136:refnum<k15>, "error out"=w135:errorcluster)  [unwired: 12 in]
      n157 = call <instrlib>:"niUSRP Close Session.vi"("session handle"=w136, "error in (no error)"=w135) -> ()  [unwired: 13 in, 1 out]
      n158 = call <instrlib>:"niUSRP Close Session.vi"("session handle"=w148, "error in (no error)"=w149) -> ()  [unwired: 13 in, 1 out]
      n159 = call "IMAQ Dispose"("Image"=w94) -> ("error out"=w95:errorcluster)  [unwired: 2 in, 3 out]
      n160 = call <vilib>:"Simple Error Handler.vi"("error in (no error)"=w95) -> ()  [unwired: 1 in, 8 out]
      n161 = call <vilib>:"IMAQdx Close Camera.vi"("error in"=w82, "Session In"=w83) -> ("error out"=w86:errorcluster)  [unwired: 9 in]
      n162 = call "IMAQ Dispose"("Image"=w84, "error in (no error)"=w86) -> ("error out"=w88:errorcluster)  [unwired: 1 in, 3 out]
      n163 = Initialize Array(cdb 0.0+0.0i, 4096 ("dimension size")) -> (w111:cdb[])
      n164 = while {
        tunnel: w150 -> [w504]
        shift-right: [w501] -> _
        shift-left: errorcluster {"status"=FALSE, "code"=0, "source"=""} ("error out") -> [w507]
        tunnel: w145 -> [w500]
        shift-right: [w499] -> _
        shift-left: errorcluster {"status"=FALSE, "code"=0, "source"=""} ("error out") -> [w498]
        tunnel: w116 -> [w496]
        tunnel: w119 -> [w495]
        tunnel: w118 -> [w494]
        tunnel: w111 -> [w493]
        i -> [w492]
        stop <- w497 stop-if-true
        n165 = Greater Or Equal?(x=w492, y=100) -> (x >= y?=w489:bool)
        n166 = Get Queue Status(queue=w504, error in (no error)=w507) -> (queue out=w502:refnum<queue>, error out=w503:errorcluster, # elements in queue=w506:i32)  [unwired: 1 in, 5 out]
        n167 = Not Equal To 0?(x=w506) -> (x != 0?=w505:bool)
        n168 = And(x=w505, y=w489) -> (x .and. y?=w490:bool)
        n169 = case shown="True" w490 {
          tunnel: w503 -> [w509 w552]
          tunnel: w502 -> [_ w551]
          tunnel: [w509 w550] -> w501
          tunnel: w500 -> [_ w545]
          tunnel: [w508 w544] -> w499
          tunnel: w498 -> [w508 w543]
          tunnel: w496 -> [_ w540]
          tunnel: w495 -> [_ w539]
          tunnel: w494 -> [_ w538]
          tunnel: w493 -> [_ w528]
          frame False {
          }
          frame True {
            # "length"
            # "Waveform \nGenerator"
            n170 = Dequeue Element(queue=w551, error in (no error)=w552) -> (element=w512:i16[], error out=w550:errorcluster)  [unwired: 1 in, 2 out]
            n171 = Unbundle(w540) -> ("samples per symbol (16)"=w534:i32, "symbol map"=w527:cdb[])  [unwired: 1 out]
            n172 = Array Size(array=w512) -> (size(s)=w536:i32)
            n173 = Quotient & Remainder(x=w536, y=8) -> (floor(x/y)=w516:i32)  [unwired: 1 out]
            n174 = To Unsigned Word Integer(number=w516) -> (unsigned 16bit integer=w535:u16)
            n175 = Number To Boolean Array(number=w535) -> (Boolean array=w549:bool[])
            n176 = Reshape Array(w549, 2 ("dimension size"), 8 ("dimension size")) -> (w546:bool[][])
            n177 = for {
              tunnel: w546 -> [w555] mode=indexing
              tunnel: [w553] -> w537 mode=indexing
              n178 = Boolean Array To Number(Boolean array=w555) -> (number=w554:u32)
              n179 = To Unsigned Byte Integer(number=w554) -> (unsigned 8bit integer=w553:u8)
            }
            n180 = Initialize Array(u8 0, 128 ("dimension size")) -> (w511:u8[])
            n181 = Build Array (concatenate)(u8[] [53, 187, 37, 71, 79, 49, 4, 63] ("Array 2"), w537, w537) -> (w542:u8[])
            n182 = call "tx_pduGen.vi"("byte array"=w542) -> ("packet bits length"=→"packet bits length":i32, "pdu"=w513:i32[])  [unwired: 3 in]
            n183 = Build Array (concatenate)(w513, w512, w511) -> (w510:i32[])
            n184 = call "sub_bits_to_symbols.vi"("symbol map"=w527, "bits"=w510) -> ("symbols"=w526:cdb[])  [unwired: 9 in]
            n185 = Build Array (concatenate)(w526, w528) -> (w524:cdb[])
            n186 = call-poly <vilib>:"MT Pulse Shaping Filter.vi"("symbols"=w524, "pulse shaping filter coefficients"=w539, "samples per symbol (16)"=w534, "symbol rate (Hz)"=w538, "reset? (T)"=FALSE) -> ("output complex waveform"=w533:T8)  [unwired: 9 in, 1 out]
            n187 = Divide(x="Transmit power (db)", y=20.0) -> (x/y=w521:dbl)
            n188 = Unbundle(w533) -> ("t0"=w532:dbl, "dt"=w531:dbl, "Y"=w519:cdb[])
            n189 = Power Of 10(x=w521) -> (10^x=w520:dbl)
            n190 = Multiply(x=w519, y=w520) -> (x*y=w518:cdb[])
            n191 = Bundle(cluster=w533, "t0"=w532, "dt"=w531, "Y"=w518) -> (w530:T8)
            n192 = Enqueue Element(queue=w545, element=w530, error in (no error)=w543) -> (error out=w544:errorcluster)  [unwired: 1 in, 2 out]
          }
        }
        n193 = global read "var_stop.vi" "system stop"() -> (w497:bool)
      }
      n194 = Unbundle By Name(w88) -> ("source"=w87:string)
      n195 = call <vilib>:"Simple Error Handler.vi"("error source (\" \")"=w87, "error in (no error)"=w88) -> ("error out"=→"error out":errorcluster)  [unwired: 3 in, 4 out]
    }
    frame Error {
    }
  }
